vi "ZS-480-CRC.vi"(11 "命令字符串":string) -> (3 "校验码":string)   [LabVIEW 2017]
uses:
  <vilib>/regexp/Match Regular Expression.xnode
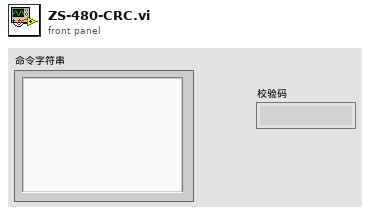
[diagram p1: front panel]
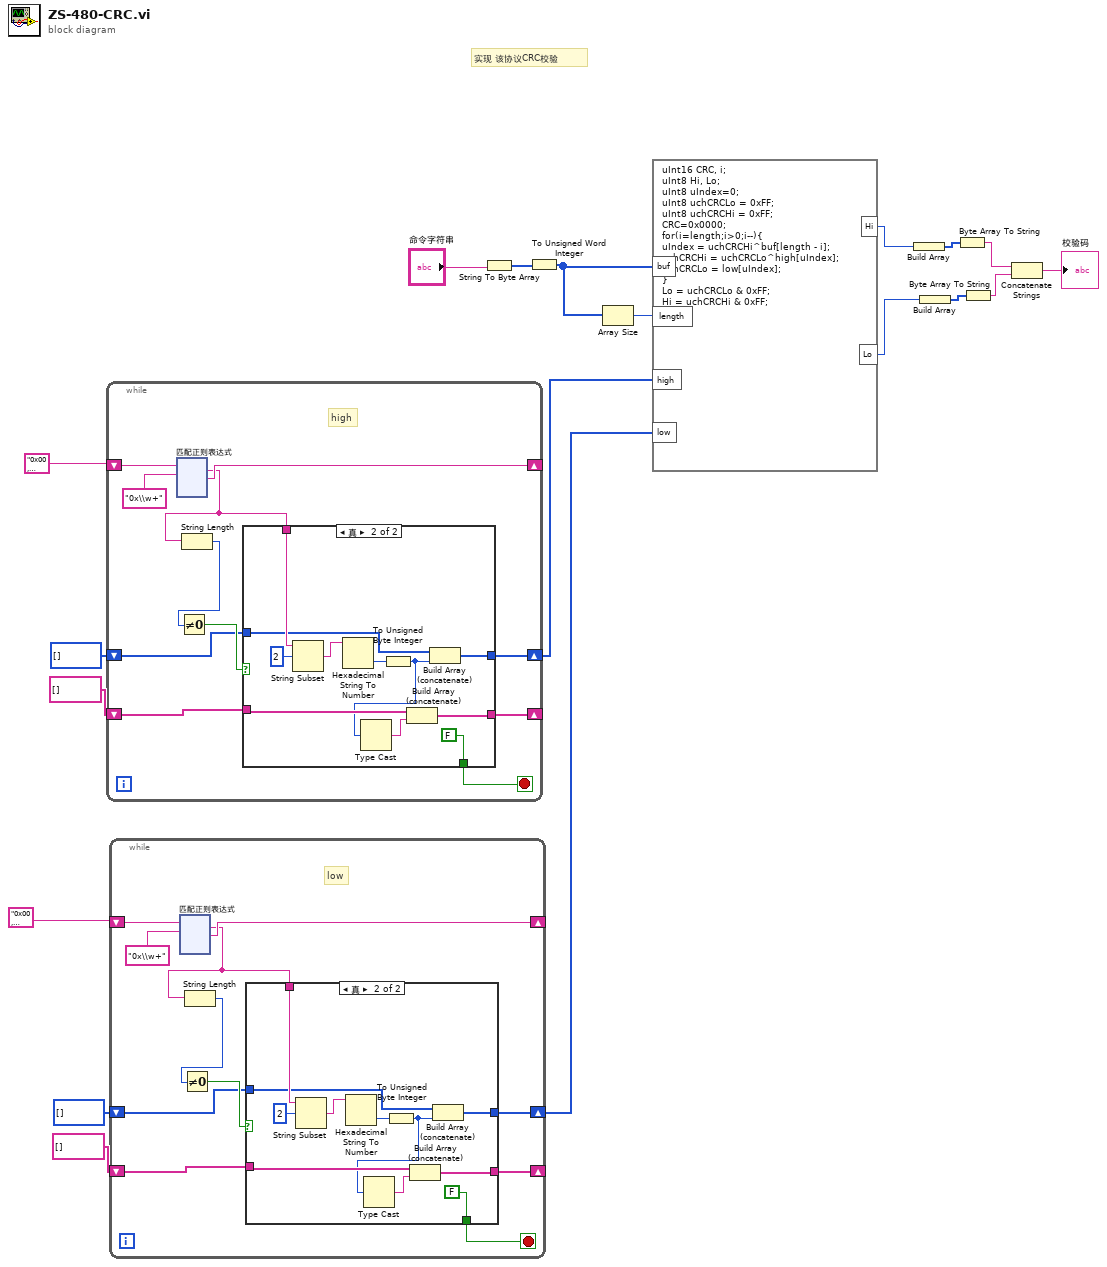
[diagram p0: block diagram]
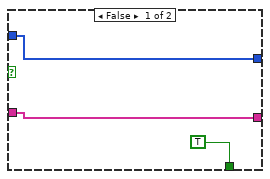
[diagram p2: hidden frame]
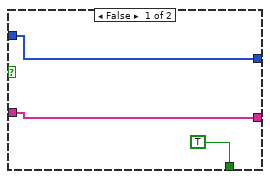
[diagram p3: hidden frame]
diagram:
  # "实现 该协议CRC校验"
  n1 = while {
    shift-right: [w29] -> _
    shift-left: "0x00, 0xC1, 0x81, 0x40, 0x01, 0xC0, 0x80, 0x41, 0x01, 0xC0, 0x80, 0x41,\n\t0x00, 0xC1, 0x81, 0x40, 0x01, 0xC0, 0x80, 0x41, 0x00, 0xC1, 0x81, 0x40,\n\t0x00, 0xC1, 0x81, 0x40, 0x01, 0xC0, 0x80, 0x41, 0x01, 0xC0, 0x80, 0x41,\n\t0x00, 0xC1, 0x81, 0x40, 0x00, 0xC1, 0x81, 0x40, 0x01, 0xC0, 0x80, 0x41,\n\t0x00, 0xC1, 0x81, 0x40, 0x01, 0xC0, 0x80, 0x41, 0x01, 0xC0, 0x80, 0x41,\n\t0x00, 0xC1, 0x81, 0x40, 0x01, 0xC0, 0x80, 0x41, 0x00, 0xC1, 0x81, 0x40,\n\t0x00, 0xC1, 0x81, 0x40, 0x01, 0xC0, 0x80, 0x41, 0x00, 0xC1, 0x81, 0x40,\n\t0x01, 0xC0, 0x80, 0x41, 0x01, 0xC0, 0x80, 0x41, 0x00, 0xC1, 0x81, 0x40,\n\t0x00, 0xC1, 0x81, 0x40, 0x01, 0xC0, 0x80, 0x41, 0x01, 0xC0, 0x80, 0x41,\n\t0x00, 0xC1, 0x81, 0x40, 0x01, 0xC0, 0x80, 0x41, 0x00, 0xC1, 0x81, 0x40,\n\t0x00, 0xC1, 0x81, 0x40, 0x01, 0xC0, 0x80, 0x41, 0x01, 0xC0, 0x80, 0x41,\n\t0x00, 0xC1, 0x81, 0x40, 0x00, 0xC1, 0x81, 0x40, 0x01, 0xC0, 0x80, 0x41,\n\t0x00, 0xC1, 0x81, 0x40, 0x01, 0xC0, 0x80, 0x41, 0x01, 0xC0, 0x80, 0x41,\n\t0x00, 0xC1, 0x81, 0x40, 0x00, 0xC1, 0x81, 0x40, 0x01, 0xC0, 0x80, 0x41,\n\t0x01, 0xC0, 0x80, 0x41, 0x00, 0xC1, 0x81, 0x40, 0x01, 0xC0, 0x80, 0x41,\n\t0x00, 0xC1, 0x81, 0x40, 0x00, 0xC1, 0x81, 0x40, 0x01, 0xC0, 0x80, 0x41,\n\t0x00, 0xC1, 0x81, 0x40, 0x01, 0xC0, 0x80, 0x41, 0x01, 0xC0, 0x80, 0x41,\n\t0x00, 0xC1, 0x81, 0x40, 0x01, 0xC0, 0x80, 0x41, 0x00, 0xC1, 0x81, 0x40,\n\t0x00, 0xC1, 0x81, 0x40, 0x01, 0xC0, 0x80, 0x41, 0x01, 0xC0, 0x80, 0x41,\n\t0x00, 0xC1, 0x81, 0x40, 0x00, 0xC1, 0x81, 0x40, 0x01, 0xC0, 0x80, 0x41,\n\t0x00, 0xC1, 0x81, 0x40, 0x01, 0xC0, 0x80, 0x41, 0x01, 0xC0, 0x80, 0x41,\n\t0x00, 0xC1, 0x81, 0x40" -> [w30]
    shift-right: [w25] -> _
    shift-left: string[] [] -> [w24]
    shift-right: [w23] -> w7
    shift-left: i8[] [] -> [w22]
    stop <- w26 stop-if-true
    # "high"
    n2 = xnode "匹配正则表达式"("输入字符串"=w30, "正则表达式"="0x\\w+") -> ("所有匹配"=w21:string, "匹配之后"=w29:string)  [unwired: 4 in, 3 out]
    n3 = String Length(string=w21) -> (length=w28:i32)
    n4 = Not Equal To 0?(x=w28) -> (x != 0?=w27:bool)
    n5 = case shown="真" w27 {
      tunnel: [w32 w40] -> w25
      tunnel: w21 -> [_ w42]
      tunnel: [TRUE FALSE] -> w26
      tunnel: w24 -> [w32 w39]
      tunnel: [w31 w37] -> w23
      tunnel: w22 -> [w31 w36]
      frame False {
      }
      frame True {
        n6 = String Subset(string=w42, offset (0)=2 ("偏移量(0)")) -> (substring=w43:string)  [unwired: 1 in]
        n7 = Hexadecimal String To Number(string=w43) -> (number=w35:u32)  [unwired: 2 in, 1 out]
        n8 = To Unsigned Byte Integer(number=w35) -> (unsigned 8bit integer=w34:u8)
        n9 = Type Cast(x=w34) -> (*(type *) &x=w38:string)  [unwired: 1 in]
        n10 = Build Array (concatenate)(w39, w38) -> (w40:string[])
        n11 = Build Array (concatenate)(w36, w34) -> (w37:u8[])
      }
    }
  }
  n12 = while {
    shift-right: [w168] -> _
    shift-left: "0x00, 0xC0, 0xC1, 0x01, 0xC3, 0x03, 0x02, 0xC2, 0xC6, 0x06, 0x07, 0xC7,\n\t0x05, 0xC5, 0xC4, 0x04, 0xCC, 0x0C, 0x0D, 0xCD, 0x0F, 0xCF, 0xCE, 0x0E,\n\t0x0A, 0xCA, 0xCB, 0x0B, 0xC9, 0x09, 0x08, 0xC8, 0xD8, 0x18, 0x19, 0xD9,\n\t0x1B, 0xDB, 0xDA, 0x1A, 0x1E, 0xDE, 0xDF, 0x1F, 0xDD, 0x1D, 0x1C, 0xDC,\n\t0x14, 0xD4, 0xD5, 0x15, 0xD7, 0x17, 0x16, 0xD6, 0xD2, 0x12, 0x13, 0xD3,\n\t0x11, 0xD1, 0xD0, 0x10, 0xF0, 0x30, 0x31, 0xF1, 0x33, 0xF3, 0xF2, 0x32,\n\t0x36, 0xF6, 0xF7, 0x37, 0xF5, 0x35, 0x34, 0xF4, 0x3C, 0xFC, 0xFD, 0x3D,\n\t0xFF, 0x3F, 0x3E, 0xFE, 0xFA, 0x3A, 0x3B, 0xFB, 0x39, 0xF9, 0xF8, 0x38,\n\t0x28, 0xE8, 0xE9, 0x29, 0xEB, 0x2B, 0x2A, 0xEA, 0xEE, 0x2E, 0x2F, 0xEF,\n\t0x2D, 0xED, 0xEC, 0x2C, 0xE4, 0x24, 0x25, 0xE5, 0x27, 0xE7, 0xE6, 0x26,\n\t0x22, 0xE2, 0xE3, 0x23, 0xE1, 0x21, 0x20, 0xE0, 0xA0, 0x60, 0x61, 0xA1,\n\t0x63, 0xA3, 0xA2, 0x62, 0x66, 0xA6, 0xA7, 0x67, 0xA5, 0x65, 0x64, 0xA4,\n\t0x6C, 0xAC, 0xAD, 0x6D, 0xAF, 0x6F, 0x6E, 0xAE, 0xAA, 0x6A, 0x6B, 0xAB,\n\t0x69, 0xA9, 0xA8, 0x68, 0x78, 0xB8, 0xB9, 0x79, 0xBB, 0x7B, 0x7A, 0xBA,\n\t0xBE, 0x7E, 0x7F, 0xBF, 0x7D, 0xBD, 0xBC, 0x7C, 0xB4, 0x74, 0x75, 0xB5,\n\t0x77, 0xB7, 0xB6, 0x76, 0x72, 0xB2, 0xB3, 0x73, 0xB1, 0x71, 0x70, 0xB0,\n\t0x50, 0x90, 0x91, 0x51, 0x93, 0x53, 0x52, 0x92, 0x96, 0x56, 0x57, 0x97,\n\t0x55, 0x95, 0x94, 0x54, 0x9C, 0x5C, 0x5D, 0x9D, 0x5F, 0x9F, 0x9E, 0x5E,\n\t0x5A, 0x9A, 0x9B, 0x5B, 0x99, 0x59, 0x58, 0x98, 0x88, 0x48, 0x49, 0x89,\n\t0x4B, 0x8B, 0x8A, 0x4A, 0x4E, 0x8E, 0x8F, 0x4F, 0x8D, 0x4D, 0x4C, 0x8C,\n\t0x44, 0x84, 0x85, 0x45, 0x87, 0x47, 0x46, 0x86, 0x82, 0x42, 0x43, 0x83,\n\t0x41, 0x81, 0x80, 0x40" -> [w169]
    shift-right: [w164] -> _
    shift-left: string[] [] -> [w163]
    shift-right: [w162] -> w6
    shift-left: i8[] [] -> [w161]
    stop <- w165 stop-if-true
    # "low"
    n13 = xnode "匹配正则表达式"("输入字符串"=w169, "正则表达式"="0x\\w+") -> ("所有匹配"=w160:string, "匹配之后"=w168:string)  [unwired: 4 in, 3 out]
    n14 = String Length(string=w160) -> (length=w167:i32)
    n15 = Not Equal To 0?(x=w167) -> (x != 0?=w166:bool)
    n16 = case shown="真" w166 {
      tunnel: [w171 w179] -> w164
      tunnel: w160 -> [_ w181]
      tunnel: [TRUE FALSE] -> w165
      tunnel: w163 -> [w171 w178]
      tunnel: [w170 w176] -> w162
      tunnel: w161 -> [w170 w175]
      frame False {
      }
      frame True {
        n17 = String Subset(string=w181, offset (0)=2 ("偏移量(0)")) -> (substring=w182:string)  [unwired: 1 in]
        n18 = Hexadecimal String To Number(string=w182) -> (number=w174:u32)  [unwired: 2 in, 1 out]
        n19 = To Unsigned Byte Integer(number=w174) -> (unsigned 8bit integer=w173:u8)
        n20 = Type Cast(x=w173) -> (*(type *) &x=w177:string)  [unwired: 1 in]
        n21 = Build Array (concatenate)(w178, w177) -> (w179:string[])
        n22 = Build Array (concatenate)(w175, w173) -> (w176:u8[])
      }
    }
  }
  n23 = String To Byte Array(string="命令字符串") -> (unsigned byte array=w18:u8[])
  n24 = To Unsigned Word Integer(number=w18) -> (unsigned 16bit integer=w16:u16[])
  n25 = Array Size(array=w16) -> (size(s)=w17:i32)
  n26 = formula code="uInt16 CRC, i;\nuInt8 Hi, Lo;\nuInt8 uIndex=0;\nuInt8 uchCRCLo = 0xFF;\nuInt8 uchCRCHi = 0xFF;\nCRC=0x0000;\nfor(i=length;i>0;i--){\nuIndex = uchCRCHi^buf[length - i];\nuchCRCHi = uchCRCLo^high[uIndex];\nuchCRCLo = low[uIndex];\n}\nLo = uchCRCLo & 0xFF;\nHi = uchCRCHi & 0xFF;"("length"=w17, "buf"=w16, "high"=w7, "low"=w6) -> ("Lo"=w15:u8, "Hi"=w4:u8)
  n27 = Build Array(w4) -> (w5:u8[])
  n28 = Build Array(w15) -> (w14:u8[])
  n29 = Byte Array To String(unsigned byte array=w5) -> (string=w3:string)
  n30 = Byte Array To String(unsigned byte array=w14) -> (string=w2:string)
  n31 = Concatenate Strings(w3, w2) -> (→"校验码":string)
